vi "SEA_LOWER_LEVEL_PI_CONTROL.vi"() -> ()   [LabVIEW 2019]
uses:
  <vilib>/rvi/Emulation/niFpgaGetClockAttributes.vi
  <vilib>/rvi/Emulation/niFpgaSctlEmulationGetInTimedLoop.vi
  <vilib>/rvi/Emulation/niFpgaEmulationReportErrorSimple.vi
  <vilib>/rvi/eio/common/nirviEmuTemplateMethod_errors.vi
  <vilib>/rvi/Emulation/niFpgaCriticalErrorInLSC.vi
  <vilib>/eio/EIONode/EIONode.xnode
  <vilib>/rvi/Arithmetic/AddSubMult/XNode/nirviSatArithmetic.xnode
panel:
  in  "transparency Current Offset":sgl=2.4882812 format="%#_13g"
  in  "transparency reference":sgl
  out "transparency filtered current":sgl
  out "transparency motor Loop rate":u32
  in  "transparency motor Kp current control":sgl
  in  "transparency motor Upper bound":sgl
  in  "transparency motor Lower bound":sgl
  in  "transparency motor Ki current control":sgl
  out "transparency Motor direction":bool
  out "transparency control_ip":sgl
  in  "Position Reset transparency side":bool
  out "Position (Counts) transparency motor side":i16
  out "Acceleration (Counts/Interval) transparency motor side":i32
  out "Velocity (Counts/Interval) transparency motor side":i32
  out "Loop time (position) transparency motor side":u32
  out "Position(Radians) transparency motor side":sgl(graph)
  in  "Position Reset":bool
  out "Position (Counts) motor side":i16
  out "Acceleration (Counts/Interval) motor side":i32
  out "Velocity (Counts/Interval) motor side":i32
  out "Loop time (position) 1 motor side":u32
  out "Position(Radians) motor side":sgl(graph)
  in  "Position Reset joint side":bool
  out "Position (Counts) joint side":i16
  out "Acceleration (Counts/Interval) joint side":i32
  out "Velocity (Counts/Interval) joint side":i32
  out "Loop time (position) joint side":u32
  out "Position(Radians) joint side":sgl(graph)
  out "control_ip":sgl
  out "Motor direction":bool
  in  "Ki current control":sgl
  in  "Lower bound":sgl
  in  "Upper bound":sgl
  in  "Kp current control":sgl
  out "Loop rate":u32
  out "filtered current":sgl
  in  "Reference":sgl
  in  "Current Offset":sgl=2.4882812 format="%#_13g"
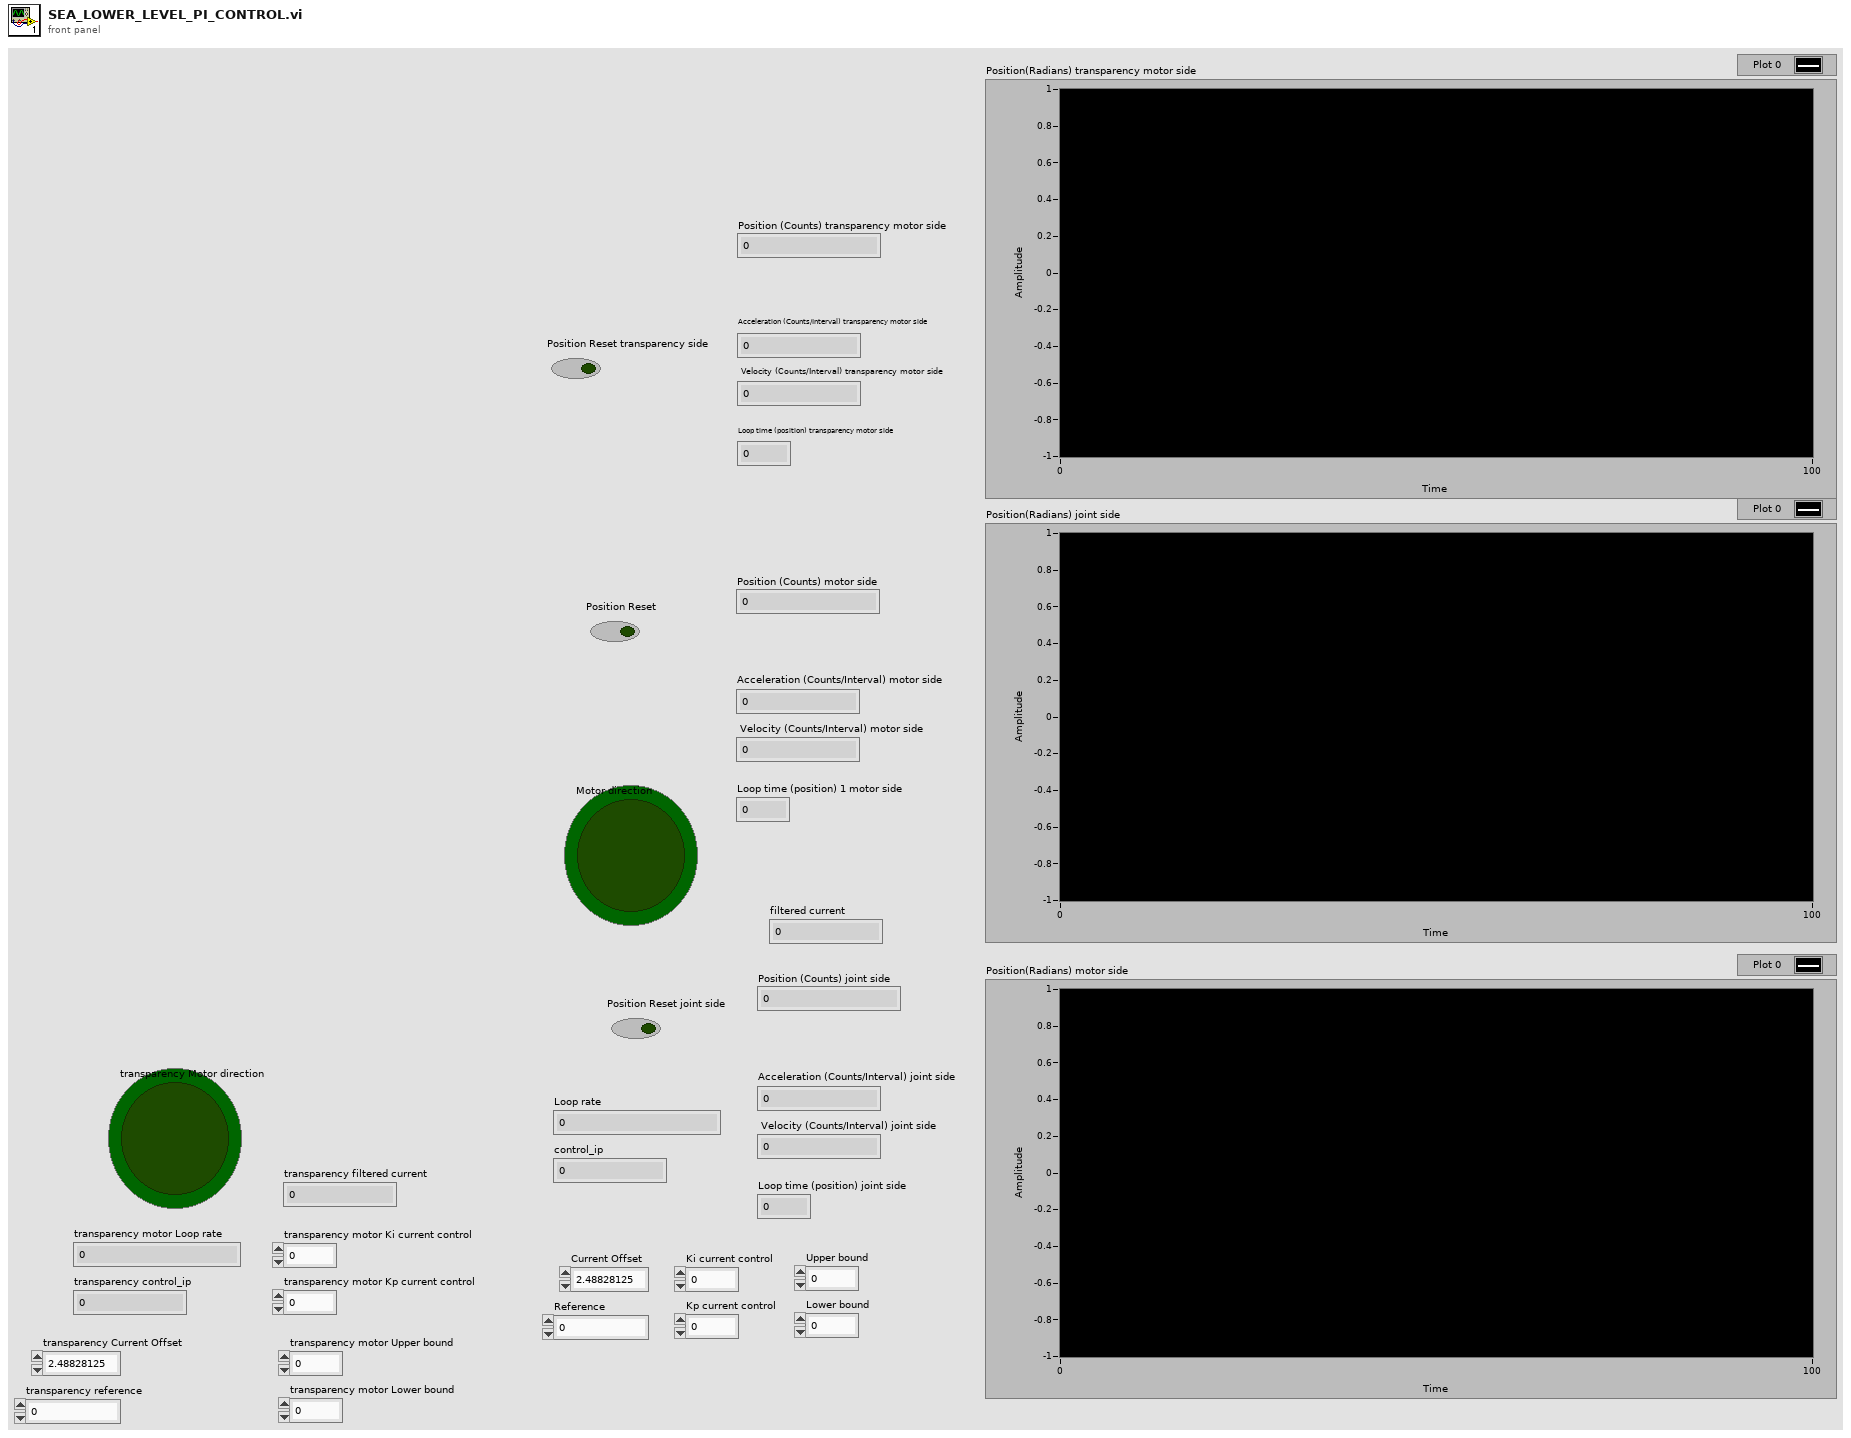
[diagram p1: front panel]
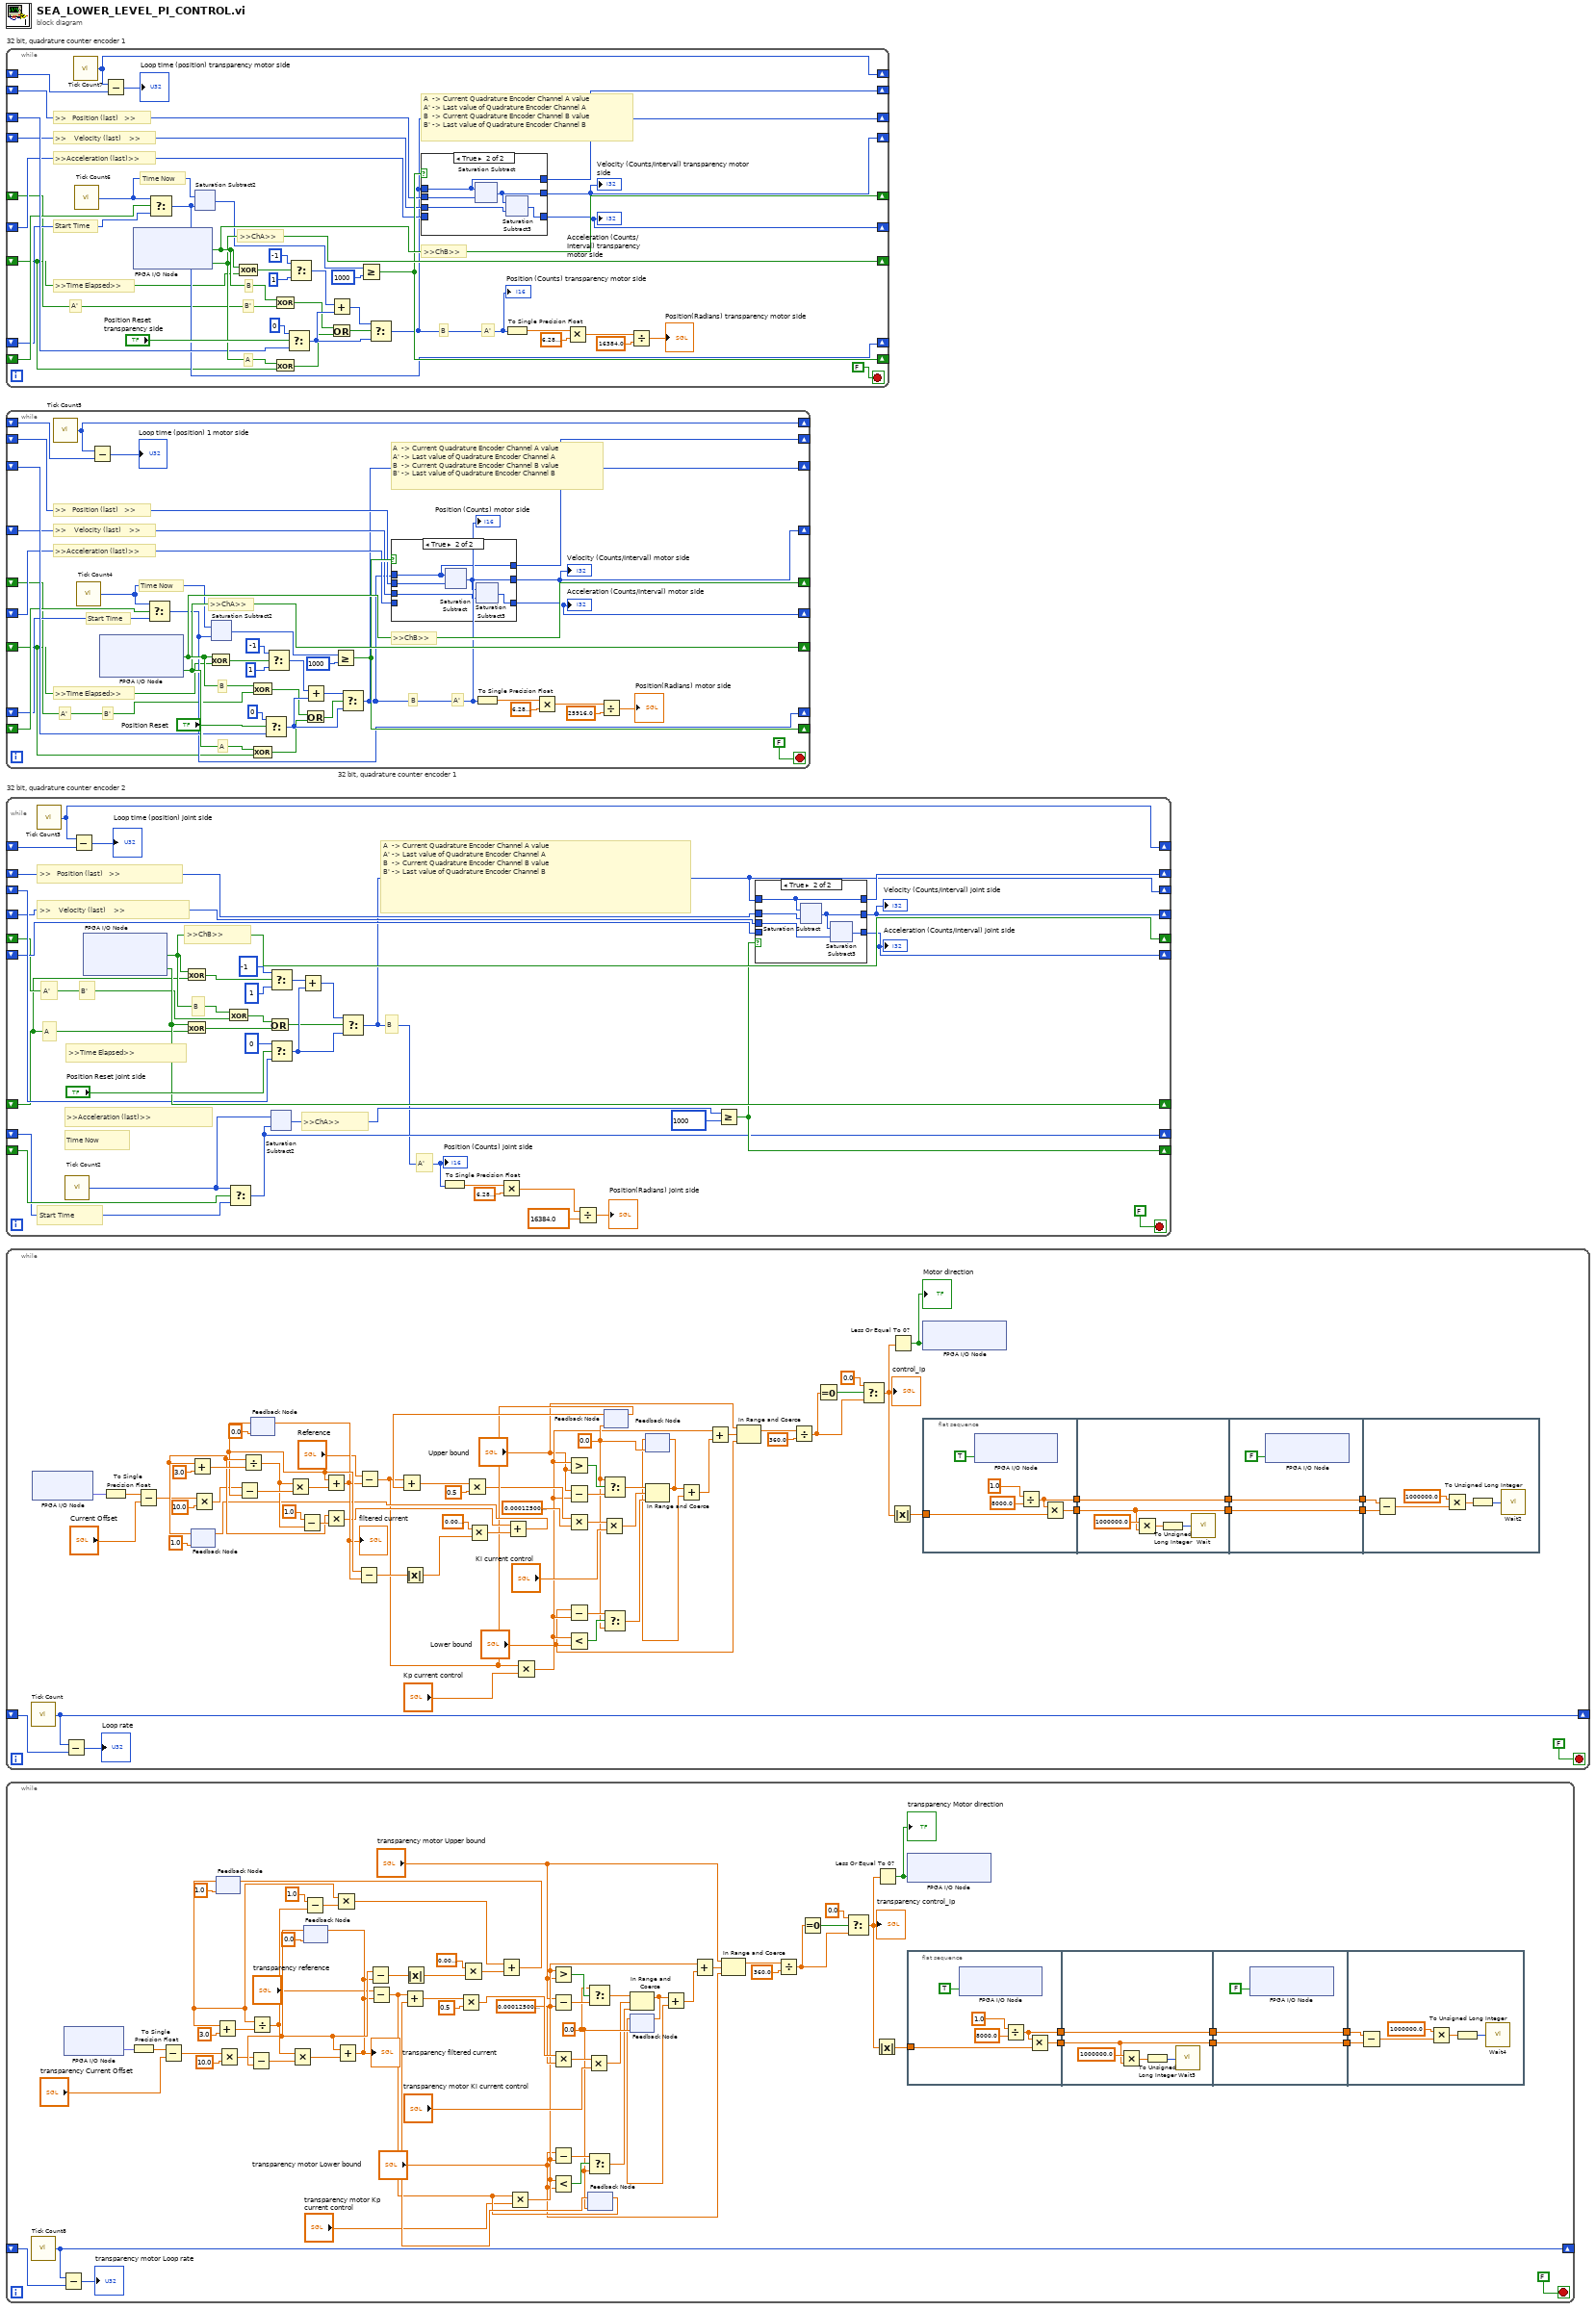
[diagram p0: block diagram]
diagram:
  n1 = while "32 bit, quadrature counter encoder 1" {
    shift-right: [w29] -> _
    shift-left: _ -> [w17]
    shift-right: [w8] -> _
    shift-left: _ -> [w26]
    shift-right: [w28] -> _
    shift-left: _ -> [w9]
    shift-right: [w23] -> _
    shift-left: _ -> [w25]
    shift-right: [w19] -> _
    shift-left: _ -> [w24]
    shift-right: [w14] -> _
    shift-left: _ -> [w13]
    shift-right: [w15] -> _
    shift-left: _ -> [w21]
    shift-right: [w16] -> _
    shift-left: _ -> [w18]
    shift-right: [w10] -> _
    shift-left: _ -> [w12]
    stop <- FALSE stop-if-true
    # "A  -> Current Quadrature Encoder Channel A value\nA' -> Last value of Quadrature Encoder Channel A\nB  -> Current Quadrature Encoder Channel B value\nB' -> Last value of Quadrature Encoder Channel B"
    # ">>Acceleration (last)>>"
    # "Start Time"
    # "A'"
    # "B"
    # "A'"
    # "A"
    # "B'"
    # "B"
    # ">>ChB>>"
    # ">>ChA>>"
    # ">>    Velocity (last)    >>"
    # ">>   Position (last)   >>"
    # "Time Now"
    # ">>Time Elapsed>>"
    n2 = call "Tick Count7"() -> ("Tick Count(Ticks)"=w10:u32)
    n3 = call "Tick Count6"() -> ("Tick Count(uSec)"=w20:u32)
    n4 = Subtract(x=w10, y=w12) -> (x-y=→"Loop time (position) transparency motor side":u32)
    n5 = xnode "FPGA I/O Node"() -> ("RMC/DIO4"=w29:bool, "RMC/DIO5"=w28:bool)  [unwired: 2 in, 2 out]
    n6 = Select(t=w20, s=w25, f=w24) -> (s? t:f=w19:u32)
    n7 = xnode ("Saturation Subtract2")("x"=w20, "y"=w19) -> ("x-y"=w22:u32)
    n8 = Exclusive Or(1:w9, 2:w29) -> (0:w30:bool)
    n9 = Exclusive Or(1:w17, 2:w29) -> (0:w31:bool)
    n10 = Exclusive Or(1:w9, 2:w28) -> (0:w32:bool)
    n11 = Select(t=0 ("32 bit"), s="Position Reset transparency side", f=w26) -> (s? t:f=w37:i32)
    n12 = Select(t=-1 ("32 bit"), s=w30, f=1 ("32 bit")) -> (s? t:f=w35:i32)
    n13 = Add(x=w35, y=w37) -> (x+y=w39:i32)
    n14 = Or(x=w31, y=w32) -> (x .or. y?=w27:bool)
    n15 = Greater Or Equal?(x=w22, y=u32 1000) -> (x >= y?=w23:bool)
    n16 = Select(t=w39, s=w27, f=w37) -> (s? t:f=w8:i32)
    "Position (Counts) transparency motor side" <- w8
    n17 = case shown="True" w23 {
      tunnel: w8 -> [_ w53]
      tunnel: w13 -> [w50 w57]
      tunnel: [w52 w56] -> w15
      tunnel: w21 -> [w52 w55]
      tunnel: [w51 w54] -> w16
      tunnel: w18 -> [w51 _]
      tunnel: [w50 w53] -> w14
      frame False {
      }
      frame True {
        n18 = xnode ("Saturation Subtract")("x"=w53, "y"=w57) -> ("x-y"=w56:i32)
        n19 = xnode ("Saturation Subtract3")("x"=w56, "y"=w55) -> ("x-y"=w54:i32)
      }
    }
    "Acceleration (Counts/Interval) transparency motor side" <- w16
    "Velocity (Counts/Interval) transparency motor side" <- w15
    n20 = To Single Precision Float(number=w8) -> (single precision float=w7:sgl)
    n21 = Multiply(x=w7, y=sgl 6.28) -> (x*y=w6:sgl)
    n22 = Divide(x=w6, y=sgl 16384.0) -> (x/y=→"Position(Radians) transparency motor side":sgl)
  }
  n23 = while "32 bit, quadrature counter encoder 1" {
    shift-right: [w122] -> _
    shift-left: _ -> [w110]
    shift-right: [w101] -> _
    shift-left: _ -> [w119]
    shift-right: [w121] -> _
    shift-left: _ -> [w102]
    shift-right: [w116] -> _
    shift-left: _ -> [w118]
    shift-right: [w112] -> _
    shift-left: _ -> [w117]
    shift-right: [w107] -> _
    shift-left: _ -> [w106]
    shift-right: [w108] -> _
    shift-left: _ -> [w114]
    shift-right: [w109] -> _
    shift-left: _ -> [w111]
    shift-right: [w103] -> _
    shift-left: _ -> [w105]
    stop <- FALSE stop-if-true
    # "A  -> Current Quadrature Encoder Channel A value\nA' -> Last value of Quadrature Encoder Channel A\nB  -> Current Quadrature Encoder Channel B value\nB' -> Last value of Quadrature Encoder Channel B"
    # ">>Acceleration (last)>>"
    # "Start Time"
    # "A'"
    # "B"
    # "A'"
    # "A"
    # "B'"
    # "B"
    # ">>ChB>>"
    # ">>ChA>>"
    # ">>    Velocity (last)    >>"
    # ">>   Position (last)   >>"
    # "Time Now"
    # ">>Time Elapsed>>"
    n24 = call "Tick Count5"() -> ("Tick Count(Ticks)"=w103:u32)
    n25 = call "Tick Count4"() -> ("Tick Count(uSec)"=w113:u32)
    n26 = Subtract(x=w103, y=w105) -> (x-y=→"Loop time (position) 1 motor side":u32)
    n27 = xnode "FPGA I/O Node"() -> ("RMC/DIO10"=w122:bool, "RMC/DIO11"=w121:bool)  [unwired: 2 in, 2 out]
    n28 = Select(t=w113, s=w118, f=w117) -> (s? t:f=w112:u32)
    n29 = Exclusive Or(1:w102, 2:w122) -> (0:w123:bool)
    n30 = xnode ("Saturation Subtract2")("x"=w113, "y"=w112) -> ("x-y"=w115:u32)
    n31 = Exclusive Or(1:w110, 2:w122) -> (0:w124:bool)
    n32 = Exclusive Or(1:w102, 2:w121) -> (0:w125:bool)
    n33 = Select(t=0 ("32 bit"), s="Position Reset", f=w119) -> (s? t:f=w130:i32)
    n34 = Select(t=-1 ("32 bit"), s=w123, f=1 ("32 bit")) -> (s? t:f=w128:i32)
    n35 = Add(x=w128, y=w130) -> (x+y=w132:i32)
    n36 = Or(x=w124, y=w125) -> (x .or. y?=w120:bool)
    n37 = Greater Or Equal?(x=w115, y=u32 1000) -> (x >= y?=w116:bool)
    n38 = Select(t=w132, s=w120, f=w130) -> (s? t:f=w101:i32)
    "Position (Counts) motor side" <- w101
    n39 = case shown="True" w116 {
      tunnel: w101 -> [_ w146]
      tunnel: w106 -> [w143 w150]
      tunnel: [w145 w149] -> w108
      tunnel: w114 -> [w145 w148]
      tunnel: [w144 w147] -> w109
      tunnel: w111 -> [w144 _]
      tunnel: [w143 w146] -> w107
      frame False {
      }
      frame True {
        n40 = xnode ("Saturation Subtract")("x"=w146, "y"=w150) -> ("x-y"=w149:i32)
        n41 = xnode ("Saturation Subtract3")("x"=w149, "y"=w148) -> ("x-y"=w147:i32)
      }
    }
    "Acceleration (Counts/Interval) motor side" <- w109
    "Velocity (Counts/Interval) motor side" <- w108
    n42 = To Single Precision Float(number=w101) -> (single precision float=w100:sgl)
    n43 = Multiply(x=w100, y=sgl 6.28) -> (x*y=w99:sgl)
    n44 = Divide(x=w99, y=sgl 25916.0) -> (x/y=→"Position(Radians) motor side":sgl)
  }
  n45 = while "32 bit, quadrature counter encoder 2" {
    shift-right: [w215] -> _
    shift-left: _ -> [w203]
    shift-right: [w194] -> _
    shift-left: _ -> [w212]
    shift-right: [w214] -> _
    shift-left: _ -> [w195]
    shift-right: [w209] -> _
    shift-left: _ -> [w211]
    shift-right: [w205] -> _
    shift-left: _ -> [w210]
    shift-right: [w200] -> _
    shift-left: _ -> [w199]
    shift-right: [w201] -> _
    shift-left: _ -> [w207]
    shift-right: [w202] -> _
    shift-left: _ -> [w204]
    shift-right: [w196] -> _
    shift-left: _ -> [w198]
    stop <- FALSE stop-if-true
    # "A  -> Current Quadrature Encoder Channel A value\nA' -> Last value of Quadrature Encoder Channel A\nB  -> Current Quadrature Encoder Channel B value\nB' -> Last value of Quadrature Encoder Channel B"
    # ">>Acceleration (last)>>"
    # "Start Time"
    # "A'"
    # "B"
    # "A'"
    # "A"
    # "B'"
    # "B"
    # ">>ChB>>"
    # ">>ChA>>"
    # ">>    Velocity (last)    >>"
    # ">>   Position (last)   >>"
    # "Time Now"
    # ">>Time Elapsed>>"
    n46 = call "Tick Count3"() -> ("Tick Count(Ticks)"=w196:u32)
    n47 = call "Tick Count2"() -> ("Tick Count(uSec)"=w206:u32)
    n48 = Subtract(x=w196, y=w198) -> (x-y=→"Loop time (position) joint side":u32)
    n49 = xnode "FPGA I/O Node"() -> ("RMC/DIO16"=w215:bool, "RMC/DIO17"=w214:bool)  [unwired: 2 in, 2 out]
    n50 = Exclusive Or(1:w195, 2:w215) -> (0:w216:bool)
    n51 = Exclusive Or(1:w195, 2:w214) -> (0:w218:bool)
    n52 = Exclusive Or(1:w203, 2:w215) -> (0:w217:bool)
    n53 = Select(t=w206, s=w211, f=w210) -> (s? t:f=w205:u32)
    n54 = Or(x=w217, y=w218) -> (x .or. y?=w213:bool)
    n55 = Select(t=-1 ("32 bit"), s=w216, f=1 ("32 bit")) -> (s? t:f=w221:i32)
    n56 = Select(t=0 ("32 bit"), s="Position Reset joint side", f=w212) -> (s? t:f=w223:i32)
    n57 = xnode ("Saturation Subtract2")("x"=w206, "y"=w205) -> ("x-y"=w208:u32)
    n58 = Add(x=w221, y=w223) -> (x+y=w225:i32)
    n59 = Select(t=w225, s=w213, f=w223) -> (s? t:f=w194:i32)
    "Position (Counts) joint side" <- w194
    n60 = To Single Precision Float(number=w194) -> (single precision float=w193:sgl)
    n61 = Multiply(x=w193, y=sgl 6.28) -> (x*y=w192:sgl)
    n62 = Divide(x=w192, y=sgl 16384.0) -> (x/y=→"Position(Radians) joint side":sgl)
    n63 = Greater Or Equal?(x=w208, y=u32 1000) -> (x >= y?=w209:bool)
    n64 = case shown="True" w209 {
      tunnel: w194 -> [_ w239]
      tunnel: w199 -> [w236 w243]
      tunnel: [w238 w242] -> w201
      tunnel: w207 -> [w238 w241]
      tunnel: [w237 w240] -> w202
      tunnel: w204 -> [w237 _]
      tunnel: [w236 w239] -> w200
      frame False {
      }
      frame True {
        n65 = xnode ("Saturation Subtract")("x"=w239, "y"=w243) -> ("x-y"=w242:i32)
        n66 = xnode ("Saturation Subtract3")("x"=w242, "y"=w241) -> ("x-y"=w240:i32)
      }
    }
    "Acceleration (Counts/Interval) joint side" <- w202
    "Velocity (Counts/Interval) joint side" <- w201
  }
  n67 = while {
    shift-right: [w317] -> _
    shift-left: _ -> [w318]
    stop <- FALSE stop-if-true
    w298 = sgl 0.0
    n68 = call "Tick Count"() -> ("Tick Count(uSec)"=w317:u32)
    n69 = xnode "FPGA I/O Node"() -> ("AI9"=w320:fxp<+/-,24,5>)  [unwired: 1 in, 1 out]
    n70 = Subtract(x=w317, y=w318) -> (x-y=→"Loop rate":u32)
    n71 = To Single Precision Float(number=w320) -> (single precision float=w319:sgl)
    n72 = Subtract(x=w319, y="Current Offset") -> (x-y=w324:sgl)
    n73 = feedback #1(sgl 1.0) -> (w333:sgl)
    n74 = Add(x=w333, y=sgl 3.0) -> (x+y=w339:sgl)
    n75 = Multiply(x=w324, y=sgl 10.0) -> (x*y=w325:sgl)
    n76 = Divide(x=w333, y=w339) -> (x/y=w336:sgl)
    n77 = feedback #2(sgl 0.0) -> (w332:sgl)
    n78 = Subtract(x=w325, y=w332) -> (x-y=w337:sgl)
    n79 = Multiply(x=w336, y=w337) -> (x*y=w338:sgl)
    n80 = Subtract(x=sgl 1.0, y=w336) -> (x-y=w335:sgl)
    n81 = Add(x=w332, y=w338) -> (x+y=w322:sgl)
    "filtered current" <- w322
    n82 = feedback-in #2(w322) -> ()
    n83 = Multiply(x=w333, y=w335) -> (x*y=w313:sgl)
    n84 = Subtract(x=w332, y=w322) -> (x-y=w334:sgl)
    n85 = Subtract(x="Reference", y=w322) -> (x-y=w310:sgl)
    n86 = Absolute Value(x=w334) -> (abs(x)=w315:sgl)
    n87 = Multiply(x=sgl 0.01, y=w315) -> (x*y=w312:sgl)
    n88 = Add(x=w313, y=w312) -> (x+y=w311:sgl)
    n89 = feedback-in #1(w311) -> ()
    n90 = Multiply(x=w310, y="Kp current control") -> (x*y=w291:sgl)
    n91 = Greater?(x=w291, y="Upper bound") -> (0:w308:bool)
    n92 = Subtract(x="Upper bound", y=w291) -> (x-y=w307:sgl)
    n93 = Subtract(x="Lower bound", y=w291) -> (x-y=w305:sgl)
    n94 = Less?(x=w291, y="Lower bound") -> (x < y?=w306:bool)
    n95 = Select(t=w298, s=w308, f=w307) -> (s? t:f=w296:sgl)
    n96 = Select(t=w305, s=w306, f=w298) -> (s? t:f=w295:sgl)
    n97 = feedback #3(w298) -> (w323:sgl)
    n98 = Add(x=w310, y=w323) -> (x+y=w304:sgl)
    n99 = Multiply(x=w304, y=sgl 0.5) -> (x*y=w302:sgl)
    n100 = Multiply(x=w302, y=sgl 0.000125) -> (x*y=w300:sgl)
    n101 = Multiply(x=w300, y="Ki current control") -> (x*y=w297:sgl)
    n102 = feedback-in #3(w310) -> ()
    n103 = feedback #4(w298) -> (w294:sgl)
    n104 = In Range and Coerce(upper limit=w296, x=w297, lower limit=w295) -> (coerced(x)=w293:sgl)  [unwired: 1 out]
    n105 = feedback-in #4(w293) -> ()
    n106 = Add(x=w293, y=w294) -> (x+y=w292:sgl)
    n107 = Add(x=w291, y=w292) -> (x+y=w290:sgl)
    n108 = In Range and Coerce(upper limit="Upper bound", x=w290, lower limit="Lower bound") -> (coerced(x)=w288:sgl)  [unwired: 1 out]
    n109 = Divide(x=w288, y=sgl 360.0) -> (x/y=w284:sgl)
    n110 = Equal To 0?(x=w284) -> (x = 0?=w286:bool)
    n111 = Select(t=sgl 0.0, s=w286, f=w284) -> (s? t:f=w281:sgl)
    "control_ip" <- w281
    n112 = Absolute Value(x=w281) -> (abs(x)=w282:sgl)
    n113 = Less Or Equal To 0?(x=w281) -> (x <= 0?=w283:bool)
    "Motor direction" <- w283
    n114 = xnode "FPGA I/O Node"("RMC/DIO18"=w283) -> ()  [unwired: 1 in, 1 out]
    n115 = flat-sequence {
      tunnel: [w351] -> w346
      tunnel: [w349] -> w345
      tunnel: w282 -> [w347]
      tunnel: w346 -> [w356]
      tunnel: [w356] -> w344
      tunnel: w345 -> [w355]
      tunnel: [w355] -> w343
      tunnel: w344 -> [w360]
      tunnel: [w360] -> w342
      tunnel: w343 -> [w359]
      tunnel: [w359] -> w341
      tunnel: w342 -> [w366]
      tunnel: w341 -> [w363]
      frame #0 {
        n116 = xnode "FPGA I/O Node"("RMC/DIO19"=TRUE) -> ()  [unwired: 1 in, 1 out]
        n117 = Divide(x=sgl 1.0, y=sgl 8000.0) -> (x/y=w349:sgl)
        n118 = Multiply(x=w349, y=w347) -> (x*y=w351:sgl)
      }
      frame #1 {
        n119 = Multiply(x=sgl 1000000.0, y=w356) -> (x*y=w354:sgl)
        n120 = To Unsigned Long Integer(number=w354) -> (unsigned 32bit integer=w353:u32)
        n121 = call "Wait"("Count(uSec)"=w353) -> ()  [unwired: 1 out]
      }
      frame #2 {
        n122 = xnode "FPGA I/O Node"("RMC/DIO19"=FALSE) -> ()  [unwired: 1 in, 1 out]
      }
      frame #3 {
        n123 = Subtract(x=w363, y=w366) -> (x-y=w365:sgl)
        n124 = Multiply(x=sgl 1000000.0, y=w365) -> (x*y=w361:sgl)
        n125 = To Unsigned Long Integer(number=w361) -> (unsigned 32bit integer=w362:u32)
        n126 = call "Wait2"("Count(uSec)"=w362) -> ()  [unwired: 1 out]
      }
    }
  }
  n127 = while {
    shift-right: [w404] -> _
    shift-left: _ -> [w405]
    stop <- FALSE stop-if-true
    w385 = sgl 0.0
    n128 = call "Tick Count8"() -> ("Tick Count(uSec)"=w404:u32)
    n129 = Subtract(x=w404, y=w405) -> (x-y=→"transparency motor Loop rate":u32)
    n130 = xnode "FPGA I/O Node"() -> ("AI0"=w407:fxp<+/-,24,5>)  [unwired: 1 in, 1 out]
    n131 = To Single Precision Float(number=w407) -> (single precision float=w406:sgl)
    n132 = Subtract(x=w406, y="transparency Current Offset") -> (x-y=w411:sgl)
    n133 = feedback #5(sgl 1.0) -> (w420:sgl)
    n134 = Add(x=w420, y=sgl 3.0) -> (x+y=w426:sgl)
    n135 = Multiply(x=w411, y=sgl 10.0) -> (x*y=w412:sgl)
    n136 = Divide(x=w420, y=w426) -> (x/y=w423:sgl)
    n137 = Subtract(x=sgl 1.0, y=w423) -> (x-y=w422:sgl)
    n138 = feedback #6(sgl 0.0) -> (w419:sgl)
    n139 = Subtract(x=w412, y=w419) -> (x-y=w424:sgl)
    n140 = Multiply(x=w423, y=w424) -> (x*y=w425:sgl)
    n141 = Multiply(x=w420, y=w422) -> (x*y=w400:sgl)
    n142 = Add(x=w419, y=w425) -> (x+y=w409:sgl)
    "transparency filtered current" <- w409
    n143 = feedback-in #6(w409) -> ()
    n144 = Subtract(x=w419, y=w409) -> (x-y=w421:sgl)
    n145 = Subtract(x="transparency reference", y=w409) -> (x-y=w397:sgl)
    n146 = Absolute Value(x=w421) -> (abs(x)=w402:sgl)
    n147 = Multiply(x=sgl 0.01, y=w402) -> (x*y=w399:sgl)
    n148 = Add(x=w400, y=w399) -> (x+y=w398:sgl)
    n149 = feedback-in #5(w398) -> ()
    n150 = Multiply(x=w397, y="transparency motor Kp current control") -> (x*y=w378:sgl)
    n151 = Greater?(x=w378, y="transparency motor Upper bound") -> (0:w395:bool)
    n152 = Subtract(x="transparency motor Upper bound", y=w378) -> (x-y=w394:sgl)
    n153 = Subtract(x="transparency motor Lower bound", y=w378) -> (x-y=w392:sgl)
    n154 = Less?(x=w378, y="transparency motor Lower bound") -> (x < y?=w393:bool)
    n155 = Select(t=w385, s=w395, f=w394) -> (s? t:f=w383:sgl)
    n156 = Select(t=w392, s=w393, f=w385) -> (s? t:f=w382:sgl)
    n157 = feedback #7(w385) -> (w410:sgl)
    n158 = Add(x=w397, y=w410) -> (x+y=w391:sgl)
    n159 = Multiply(x=w391, y=sgl 0.5) -> (x*y=w389:sgl)
    n160 = Multiply(x=w389, y=sgl 0.000125) -> (x*y=w387:sgl)
    n161 = Multiply(x=w387, y="transparency motor Ki current control") -> (x*y=w384:sgl)
    n162 = feedback-in #7(w397) -> ()
    n163 = In Range and Coerce(upper limit=w383, x=w384, lower limit=w382) -> (coerced(x)=w380:sgl)  [unwired: 1 out]
    n164 = feedback-in #8(w380) -> ()
    n165 = feedback #8(w385) -> (w381:sgl)
    n166 = Add(x=w380, y=w381) -> (x+y=w379:sgl)
    n167 = Add(x=w378, y=w379) -> (x+y=w377:sgl)
    n168 = In Range and Coerce(upper limit="transparency motor Upper bound", x=w377, lower limit="transparency motor Lower bound") -> (coerced(x)=w375:sgl)  [unwired: 1 out]
    n169 = Divide(x=w375, y=sgl 360.0) -> (x/y=w371:sgl)
    n170 = Equal To 0?(x=w371) -> (x = 0?=w373:bool)
    n171 = Select(t=sgl 0.0, s=w373, f=w371) -> (s? t:f=w368:sgl)
    "transparency control_ip" <- w368
    n172 = Absolute Value(x=w368) -> (abs(x)=w369:sgl)
    n173 = Less Or Equal To 0?(x=w368) -> (x <= 0?=w370:bool)
    "transparency Motor direction" <- w370
    n174 = xnode "FPGA I/O Node"("RMC/DIO22"=w370) -> ()  [unwired: 1 in, 1 out]
    n175 = flat-sequence {
      tunnel: [w438] -> w433
      tunnel: [w436] -> w432
      tunnel: w369 -> [w434]
      tunnel: w433 -> [w443]
      tunnel: [w443] -> w431
      tunnel: w432 -> [w442]
      tunnel: [w442] -> w430
      tunnel: w431 -> [w447]
      tunnel: [w447] -> w429
      tunnel: w430 -> [w446]
      tunnel: [w446] -> w428
      tunnel: w429 -> [w453]
      tunnel: w428 -> [w450]
      frame #0 {
        n176 = xnode "FPGA I/O Node"("RMC/DIO21"=TRUE) -> ()  [unwired: 1 in, 1 out]
        n177 = Divide(x=sgl 1.0, y=sgl 8000.0) -> (x/y=w436:sgl)
        n178 = Multiply(x=w436, y=w434) -> (x*y=w438:sgl)
      }
      frame #1 {
        n179 = Multiply(x=sgl 1000000.0, y=w443) -> (x*y=w441:sgl)
        n180 = To Unsigned Long Integer(number=w441) -> (unsigned 32bit integer=w440:u32)
        n181 = call "Wait3"("Count(uSec)"=w440) -> ()  [unwired: 1 out]
      }
      frame #2 {
        n182 = xnode "FPGA I/O Node"("RMC/DIO21"=FALSE) -> ()  [unwired: 1 in, 1 out]
      }
      frame #3 {
        n183 = Subtract(x=w450, y=w453) -> (x-y=w452:sgl)
        n184 = Multiply(x=sgl 1000000.0, y=w452) -> (x*y=w448:sgl)
        n185 = To Unsigned Long Integer(number=w448) -> (unsigned 32bit integer=w449:u32)
        n186 = call "Wait4"("Count(uSec)"=w449) -> ()  [unwired: 1 out]
      }
    }
  }
